vi "Model - Init.vi"(8 "error in (no error)":errorcluster) -> (0 "error out":errorcluster, 3 "View Model":T1)   [LabVIEW 2017]
doc: "Initialize all ueser events and DVRs of View Model."
uses:
  Controls/View Model.ctl
  Error Handler/Controls/Error Model.ctl
  Error Handler/Controls/Error Data.ctl
  Error Handler/Controls/Error Type.ctl
  Controls/Shared Model.ctl
  Configuration/Controls/Config Model.ctl
  Configuration/Controls/Config CMD.ctl
  Configuration/Controls/Config Data.ctl
  ATM Controller/Controls/Controller Model.ctl
  ATM Controller/Controls/Controller Overhead.ctl
  ATM Controller/Controls/Controller States.ctl
  ATM Controller/Controls/Controller Message Data.ctl
  ATM Controller/Controls/Controller Message Name.ctl
  ATM Controller/Controls/Controller CMD.ctl
  Views/User Console View/Controls/User Console - Transaction Enum.ctl
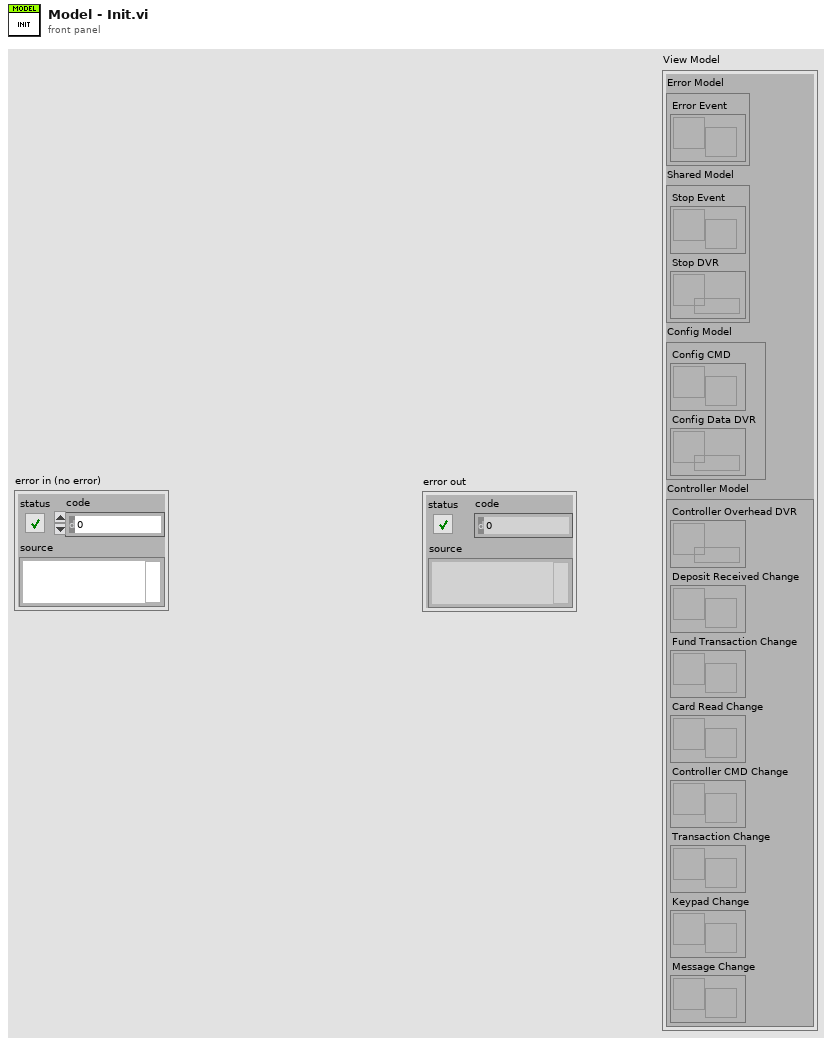
[diagram p1: front panel]
types:
  T1 = typedef "View Model.ctl" = cluster{"Error Model":T2, "Shared Model":T3, "Config Model":T4, "Controller Model":T5}
  T2 = typedef "Error Model.ctl" = cluster{"Error Event":refnum<user-event>}
  T3 = typedef "Shared Model.ctl" = cluster{"Stop Event":refnum<user-event>, "Stop DVR":refnum<data-value>}
  T4 = typedef "Config Model.ctl" = cluster{"Config CMD":refnum<user-event>, "Config Data DVR":refnum<data-value>}
  T5 = typedef "Controller Model.ctl" = cluster{"Controller Overhead DVR":refnum<data-value>, "Deposit Received Change":refnum<user-event>, "Fund Transaction Change":refnum<user-event>, "Card Read Change":refnum<user-event>, "Controller CMD Change":refnum<user-event>, "Transaction Change":refnum<user-event>, "Keypad Change":refnum<user-event>, "Message Change":refnum<user-event>}
  T6 = typedef "User Console - Transaction Enum.ctl" = enum16{"Balance Inquiry", "Deposit", "Withdrawal", "Fat Cash", "New Transaction", "Terminate Session"}
  T7 = typedef "Controller Message Data.ctl" = cluster{"Transaction":string, "Message":string, "Card Read":bool, "Message Name":T8}
  T8 = typedef "Controller Message Name.ctl" = enum16{"Welcome", "Login", "Idle", "Invalid Login", "Terminate", "Deposit", "Withdrawal", "Fast Cash", "Withdrawal Complete", "Withdrawal Failed", "Balance Inquiry"}
  T9 = typedef "Controller CMD.ctl" = cluster{"Controller State":T10, "Variant":variant}
  T10 = typedef "Controller States.ctl" = enum16{"Idle", "Init", "Display Message", "Login", "Balance Inquiry", "Deposit", "Withdrawal", "Fast Cash", "Terminate"}
  T11 = typedef "Controller Overhead.ctl" = cluster{"Account found":bool, "Current State":T10, "Next State":T10, "Inactivity Time":dbl, "Account Number":dbl, "Deposit Amount":dbl, "Withdrawal Amount":dbl, "Message Data List":T7[], "Invalid login":i16}
  T12 = typedef "Config Data.ctl" = cluster{"Account Number":i32, "Balance":dbl, "First Name":string, "Last Name":string}
  T13 = typedef "Config CMD.ctl" = enum16{"Read", "Update", "Search"}
  T14 = typedef "Error Data.ctl" = cluster{"Error Type":T15, "Variant":variant}
  T15 = typedef "Error Type.ctl" = enum16{"Console Error", "Sensor Interface IO Error", "Process Step Error"}
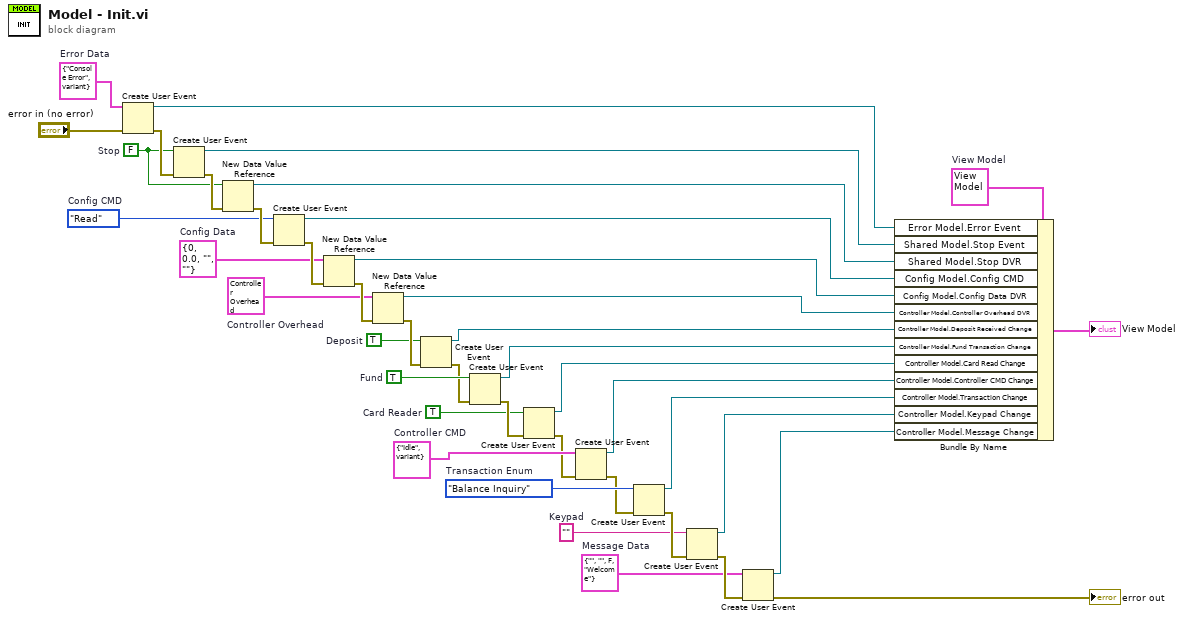
[diagram p0: block diagram]
diagram:
  w7 = ""  # Keypad
  w11 = User_Console_-_Transaction_Enum."Balance Inquiry"  # Transaction Enum
  w4 = T7 {"Transaction"="", "Message"="", "Card Read"=FALSE, "Message Name"=enum."Welcome"}  # Message Data
  w14 = T9 {"Controller State"=enum."Idle", "Variant"=variant}  # Controller CMD
  w16 = TRUE  # Card Reader
  w20 = TRUE  # Fund
  w22 = TRUE  # Deposit
  w25 = T11 {"Account found"=FALSE, "Current State"=enum."Idle", "Next State"=enum."Idle", "Inactivity Time"=0.0, "Account Number"=0.0, "Deposit Amount"=0.0, "Withdrawal Amount"=0.0, "Message Data List"=[], "Invalid login"=0}  # Controller Overhead
  w28 = T12 {"Account Number"=0, "Balance"=0.0, "First Name"="", "Last Name"=""}  # Config Data
  w31 = Config_CMD."Read"  # Config CMD
  w39 = T14 {"Error Type"=enum."Console Error", "Variant"=variant}  # Error Data
  w34 = FALSE  # Stop
  w41 = T1 {"Error Model"={"Error Event"=refnum}, "Shared Model"={"Stop Event"=refnum, "Stop DVR"=refnum}, "Config Model"={"Config CMD"=refnum, "Config Data DVR"=refnum}, "Controller Model"={"Controller Overhead DVR"=refnum, "Deposit Received Change"=refnum, "Fund Transaction Change"=refnum, "Card Read Change"=refnum, "Controller CMD Change"=refnum, "Transaction Change"=refnum, "Keypad Change"=refnum, "Message Change"=refnum}}  # View Model
  n1 = Create User Event(user event datatype=w39, error in="error in (no error)") -> (user event=w38:refnum<user-event>, error out=w37:errorcluster)
  n2 = Create User Event(user event datatype=w34, error in=w37) -> (user event=w36:refnum<user-event>, error out=w35:errorcluster)
  n3 = New Data Value Reference(data value=w34, error in=w35) -> (data value reference=w33:refnum<data-value>, error out=w32:errorcluster)
  n4 = Create User Event(user event datatype=w31, error in=w32) -> (user event=w30:refnum<user-event>, error out=w29:errorcluster)
  n5 = New Data Value Reference(data value=w28, error in=w29) -> (data value reference=w27:refnum<data-value>, error out=w26:errorcluster)
  n6 = New Data Value Reference(data value=w25, error in=w26) -> (data value reference=w24:refnum<data-value>, error out=w23:errorcluster)
  n7 = Create User Event(user event datatype=w22, error in=w23) -> (user event=w21:refnum<user-event>, error out=w19:errorcluster)
  n8 = Create User Event(user event datatype=w20, error in=w19) -> (user event=w18:refnum<user-event>, error out=w17:errorcluster)
  n9 = Create User Event(user event datatype=w16, error in=w17) -> (user event=w15:refnum<user-event>, error out=w13:errorcluster)
  n10 = Create User Event(user event datatype=w14, error in=w13) -> (user event=w12:refnum<user-event>, error out=w10:errorcluster)
  n11 = Create User Event(user event datatype=w11, error in=w10) -> (user event=w9:refnum<user-event>, error out=w8:errorcluster)
  n12 = Create User Event(user event datatype=w7, error in=w8) -> (user event=w6:refnum<user-event>, error out=w5:errorcluster)
  n13 = Create User Event(user event datatype=w4, error in=w5) -> (user event=w3:refnum<user-event>, error out=→"error out":errorcluster)
  n14 = Bundle By Name(cluster=w41, "Error Model.Error Event"=w38, "Shared Model.Stop Event"=w36, "Shared Model.Stop DVR"=w33, "Config Model.Config CMD"=w30, "Config Model.Config Data DVR"=w27, "Controller Model.Controller Overhead DVR"=w24, "Controller Model.Deposit Received Change"=w21, "Controller Model.Fund Transaction Change"=w18, "Controller Model.Card Read Change"=w15, "Controller Model.Controller CMD Change"=w12, "Controller Model.Transaction Change"=w9, "Controller Model.Keypad Change"=w6, "Controller Model.Message Change"=w3) -> (→"View Model":T1)
